vi "Fetal ECG Signal Extraction_1.vi"() -> ()   [LabVIEW 2014]
doc: "This example demonstrates how to extract fetal electrocardiogram (ECG) signals from maternal abdominal ECG signals. You obtain maternal abdominal ECG signals from obdominal leads. Maternal abdominal ECG signals contain both maternal ECG signals and fetal ECG signals. You can use an adaptive filter to extract fetal ECG signals from maternal abdominal ECG signals. To use an adaptive filter as the solution, you must obtain maternal thorax ECG signals from thorax leads as reference signals."
uses:
  <vilib>/addons/Adaptive Filters/Create/AFT Create FIR LMS (Real).vi
  <vilib>/addons/Adaptive Filters/Processing/AFT Filter Signal and Update Coefficients (Real, Array).vi
  <vilib>/addons/Adaptive Filters/NI_AdaptiveFilter.lvlib
  <vilib>/measure/NI_MABase.lvlib
panel:
  in  "sampling info":cluster{"Fs":dbl, "#s":dbl}={"Fs"=1000.0, "#s"=1000.0} {"Fs" format="%.2p"}
  in  "amplitude":dbl=1.0 format="%0.2p"
  in  "Tab Control":enum32{"Background", "ECG Signals"}(tab)
  out "Waveform Graph 3":dbl[](graph)
  out "Waveform Graph 2":dbl[](graph)
  out "Waveform Graph":dbl[](graph)
  in  "Step Size":dbl=0.45 min=0.0 step=0.01 format="%#_9f"
  in  "Filter Length":i32=40 min=2
  # "Fetal ECG signal extraction is one of adaptive noise cancellation applications. Refer to the Adaptive Noise Cancellation topic in the LabVIEW Help for more information about the background of adaptive noise cancellation. Select Help>>Show Context Help and move the cursor over the VI icon of this example for more information."
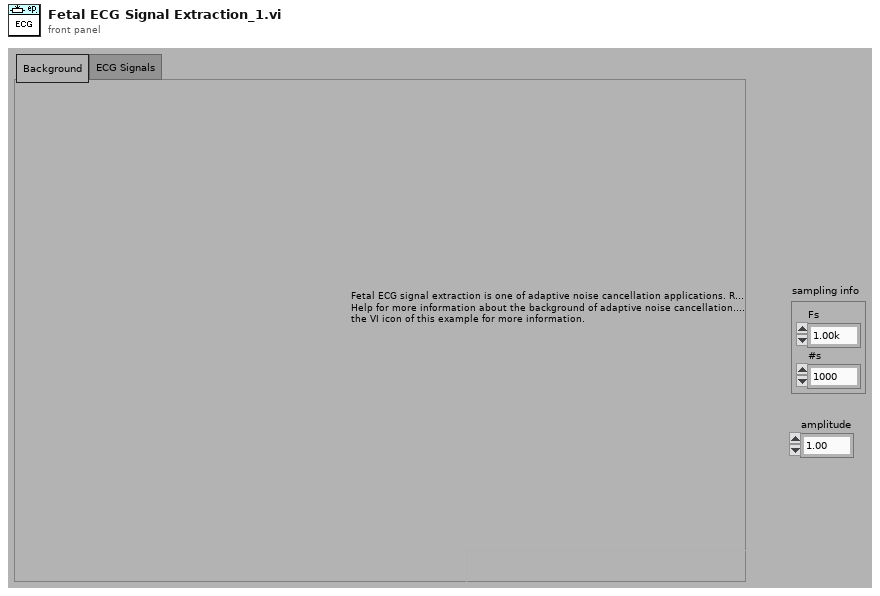
[diagram p1: front panel]
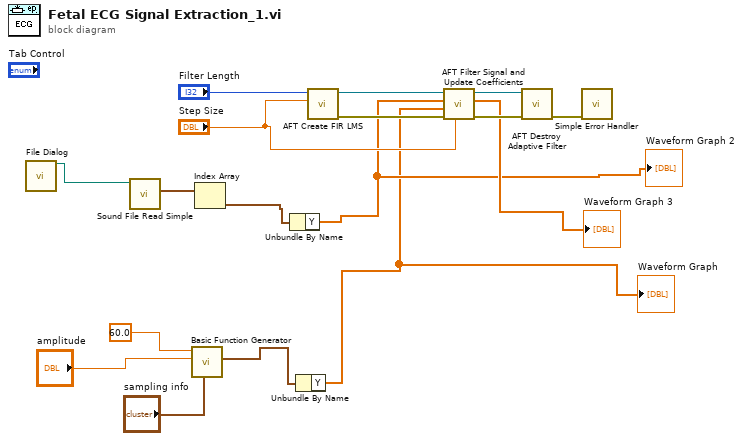
[diagram p0: block diagram]
diagram:
  n1 = call "File Dialog"() -> ("selected path"=w11:path)  [unwired: 12 in, 3 out]
  n2 = call <vilib>:"Sound File Read Simple.vi"("path"=w11) -> ("data"=w10:waveform(dbl)[])  [unwired: 7 in, 3 out]
  n3 = call <vilib>:"Basic Function Generator.vi"("sampling info"="sampling info", "amplitude"="amplitude", "frequency"=60.0) -> ("signal out"=w2:waveform(dbl))  [unwired: 6 in, 2 out]
  n4 = Index Array(array=w10) -> (element=w4:waveform(dbl))  [unwired: 1 in]
  n5 = Unbundle By Name(w4) -> ("Y"=w3:dbl[])
  "Waveform Graph 2" <- w3
  n6 = Unbundle By Name(w2) -> ("Y"=w1:dbl[])
  "Waveform Graph" <- w1
  n7 = call-poly <vilib>:"AFT Create FIR LMS.vi"("step size"="Step Size", "filter length"="Filter Length") -> ("error out"=w13:errorcluster, "adaptive filter out"=w14:refnum<k20>)  [unwired: 2 in, 6 out]
  n8 = call-poly <vilib>:"AFT Filter Signal and Update Coefficients.vi"("step size"="Step Size", "error in (no error)"=w13, "d(n)"=w1, "x(n)"=w3, "adaptive filter in"=w14) -> ("error out"=w16:errorcluster, "y(n)"=→"Waveform Graph 3":dbl[], "adaptive filter out"=w17:refnum<k20>)  [unwired: 1 in, 3 out]
  n9 = call <vilib>:"AFT Destroy Adaptive Filter.vi"("error in (no error)"=w16, "adaptive filter in"=w17) -> ("error out"=w12:errorcluster)  [unwired: 9 out]
  n10 = call <vilib>:"Simple Error Handler.vi"("error in (no error)"=w12) -> ()  [unwired: 1 in, 8 out]
